vi "Get SMO PGSQL Log Paths.vi"(5 "getAll Cluster":variant, 6 "Deprecated":bool, 7 "Default Paths":string, 8 "error in (no error)":errorcluster, 11 "Instrument in":refnum<class "Instrument.lvclass">) -> (0 "error out":errorcluster, 2 "Paths":string, 3 "Instrument out":refnum<class "Instrument.lvclass">)   [LabVIEW 2019, in "Instrument.lvlib" / "Instrument.lvclass"]
doc: "Deprecated in favor of Get SMO Database Paths.vi"
uses:
  Instrument.lvclass
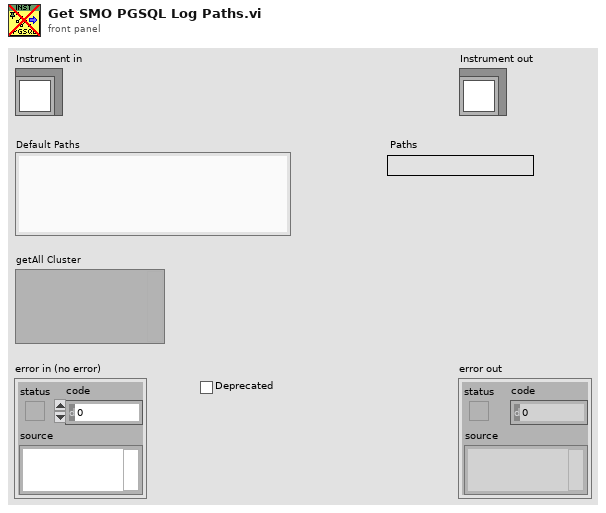
[diagram p1: front panel]
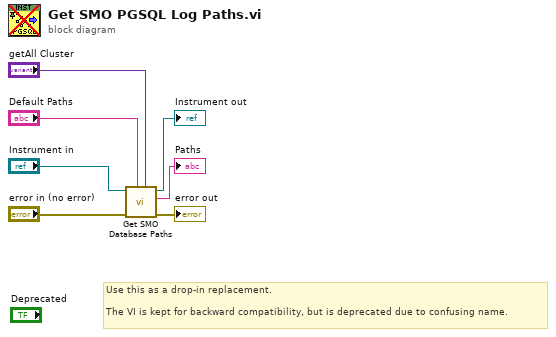
[diagram p0: block diagram]
diagram:
  # "Use this as a drop-in replacement.\n\nThe VI is kept for backward compatibility, but is deprecated due to confusing name."
  n1 = call-dynamic "Get SMO Database Paths.vi"("getAll Cluster"="getAll Cluster", "Default Paths"="Default Paths", "error in (no error)"="error in (no error)", "Instrument in"="Instrument in") -> ("error out"=→"error out":errorcluster, "Paths"=→"Paths":string, "Instrument out"=→"Instrument out":refnum<class "Instrument.lvclass">)  [unwired: 5 in]
